vi "Add Header.vi"(8 "error in":errorcluster, 9 "value":string, 10 "header":string, 11 "net-http-client in":refnum<class "net-http-client.lvclass">) -> (0 "error out":errorcluster, 3 "net-http-client out":refnum<class "net-http-client.lvclass">)   [LabVIEW 2020, in "net-http-client.lvclass"]
uses:
  net-http-client.lvclass
  net-http-client.lvclass/net-http-client.ctl
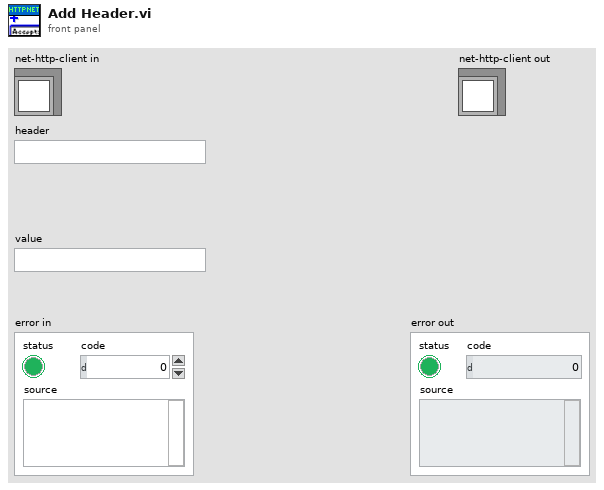
[diagram p1: front panel]
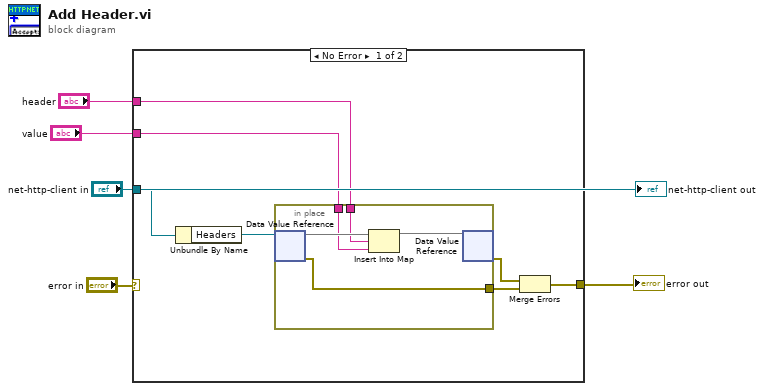
[diagram p0: block diagram]
diagram:
  n1 = case shown="No Error" "error in" {
    selector: "error in" -> [_ w18]
    tunnel: "net-http-client in" -> [w12 _]
    tunnel: "header" -> [w10 _]
    tunnel: "value" -> [w9 _]
    tunnel: [w8 w18] -> w2
    frame No Error {
      n2 = Unbundle By Name(w12) -> ("Headers"=w11:refnum<data-value>)
      n3 = in-place {
        in-place-border: w10 -> [w16]
        in-place-border: w9 -> [w15]
        in-place-border: [w14] -> w6
        n4 = in-place-dvr #1(w11) -> (w17:map{string, string}, w14:errorcluster)
        n5 = Insert Into Map(map in=w17, key=w16, value=w15) -> (map out=w13:map{string, string})  [unwired: 2 out]
        n6 = in-place-dvr #1(w13) -> (w7:errorcluster)  [unwired: 1 out]
      }
      n7 = Merge Errors(w7, w6) -> (w8:errorcluster)
    }
    frame Error {
    }
  }
  "error out" <- w2
  "net-http-client out" <- "net-http-client in"
